vi "Query Output Protection Setpoint.vi"(8 "error in (no error)":errorcluster, 11 "VISA resource name":refnum<visa-resource-name>) -> (0 "error out":errorcluster, 1 "OVC Setpoint (amps)":dbl, 2 "OVP Setpoint (volts)":dbl, 3 "VISA resource name out":refnum<visa-resource-name>, 5 "OPP Setpoint (watts)":dbl)   [LabVIEW 2018, in "XP Power PLS600.lvlib"]
doc: "Queries the present setpoint for over voltage protection (OVP), over current protection (OCP), and over power protection (OPP)."
uses:
  XP Power PLS600.lvlib
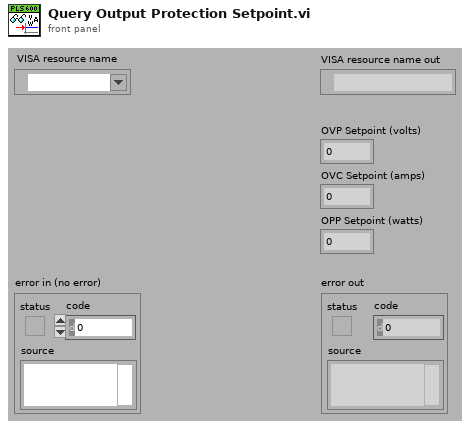
[diagram p1: front panel]
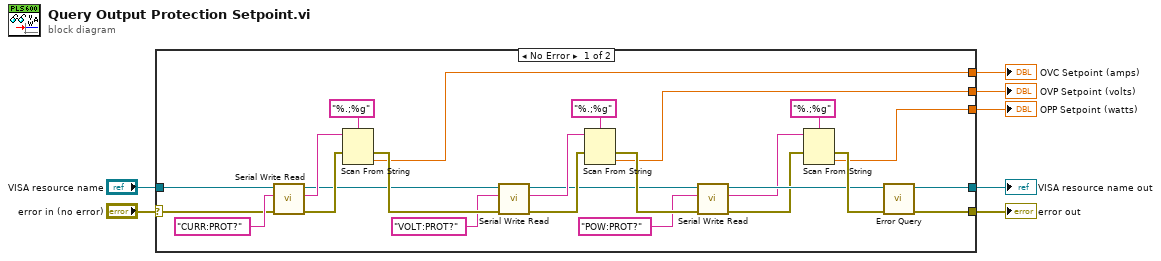
[diagram p0: block diagram]
diagram:
  n1 = case shown="No Error" "error in (no error)" {
    selector: "error in (no error)" -> [w11 w34]
    tunnel: [w32 w33] -> w7
    tunnel: [w31 w34] -> w6
    tunnel: "VISA resource name" -> [w26 w33]
    tunnel: [w10 _] -> w3
    tunnel: [w9 _] -> w2
    tunnel: [w8 _] -> w1
    frame No Error {
      n2 = call "Serial Write Read.vi"("error in (no error)"=w11, "Write Buffer"="CURR:PROT?", "VISA resource name"=w26) -> ("error out"=w23:errorcluster, "Read Buffer"=w24:string, "VISA resource name out"=w21:refnum<visa-resource-name>)  [unwired: 6 in]
      n3 = Scan From String(format string="%.;%g", input string=w24, error in=w23) -> (error out=w22:errorcluster, output 1=w10:dbl)  [unwired: 2 in, 2 out]
      n4 = call "Serial Write Read.vi"("error in (no error)"=w22, "Write Buffer"="VOLT:PROT?", "VISA resource name"=w21) -> ("error out"=w18:errorcluster, "Read Buffer"=w19:string, "VISA resource name out"=w16:refnum<visa-resource-name>)  [unwired: 6 in]
      n5 = Scan From String(format string="%.;%g", input string=w19, error in=w18) -> (error out=w17:errorcluster, output 1=w9:dbl)  [unwired: 2 in, 2 out]
      n6 = call "Serial Write Read.vi"("error in (no error)"=w17, "Write Buffer"="POW:PROT?", "VISA resource name"=w16) -> ("error out"=w12:errorcluster, "Read Buffer"=w13:string, "VISA resource name out"=w14:refnum<visa-resource-name>)  [unwired: 6 in]
      n7 = Scan From String(format string="%.;%g", input string=w13, error in=w12) -> (error out=w27:errorcluster, output 1=w8:dbl)  [unwired: 2 in, 2 out]
      n8 = call "Error Query.vi"("error in (no error)"=w27, "VISA resource name"=w14) -> ("error out"=w31:errorcluster, "VISA resource name out"=w32:refnum<visa-resource-name>)  [unwired: 6 in, 2 out]
    }
    frame Error {
    }
  }
  "VISA resource name out" <- w7
  "error out" <- w6
  "OVC Setpoint (amps)" <- w3
  "OVP Setpoint (volts)" <- w2
  "OPP Setpoint (watts)" <- w1
